vi "ch_to_cellement.vi"(7 "chtree config":T1={"ch"=[{"String"="通道名称", "use"=TRUE, "display"=0, "Enum"=enum."Chname"}, {"String"="使用", "use"=TRUE, "display"=0, "Enum"=enum."USE"}, {"String"="频率", "use"=TRUE, "display"=0, "Enum"=enum."fre"}, {"String"="范围", "use"=FALSE, "display"=0, "Enum"=enum."range"}, {"String"="传感器", "use"=TRUE, "display"=0, "Enum"=enum."senNO"}, {"String"="物理量", "use"=TRUE, "display"=0, "Enum"=enum."PHname"}, {"String"="单位", "use"=TRUE, "display"=0, "Enum"=enum."unit"}, {"String"="校准类型", "use"=FALSE, "display"=0, "Enum"=enum."CALclass"}, {"String"="校准系数", "use"=FALSE, "display"=0, "Enum"=enum."K"}, {"String"="校准偏量", "use"=TRUE, "display"=0, "Enum"=enum."K"}, {"String"="报警", "use"=TRUE, "display"=0, "Enum"=enum."Alrm"}, {"String"="", "use"=FALSE, "display"=0, "Enum"=enum."CNO."}, {"String"="", "use"=FALSE, "display"=0, "Enum"=enum."CNO."}], "displya num"=1, "range value"=["0~10V", "0~5V", "±10V", "±5V", "", "", "", "", "", "", "", "", "", "", "", "", "", "", "", ""], "Etype"=["电压", "电流", "电阻", "±5V", "", "", "", "", "", "", "", "", "", "", "", "", "", "", "", ""], "CLASS"=[]}, 10 "element":T3 {"display" format="%b"}) -> (2 "chtree cell Array":string[](array[string]))   [LabVIEW 2011]
uses:
  singlechtype.ctl
  chtype.ctl
  config table enum.ctl
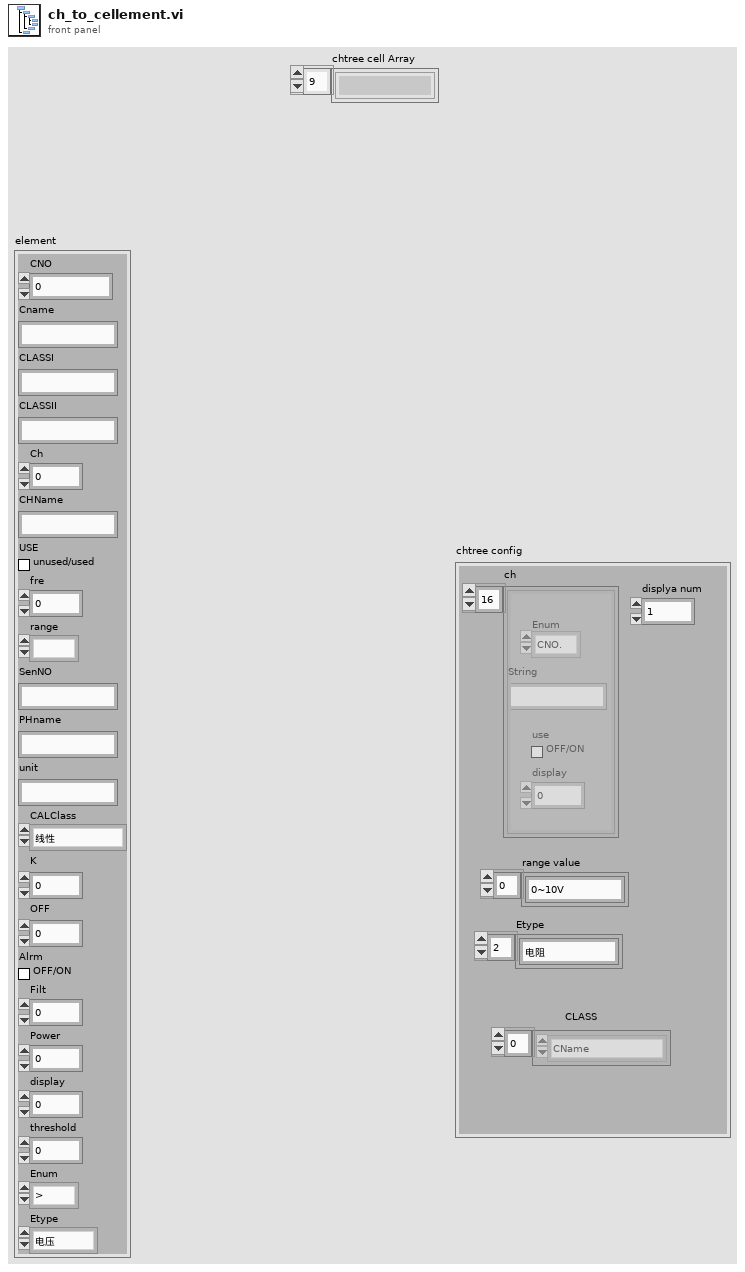
[diagram p1: front panel]
types:
  T1 = typedef "chtype.ctl" = cluster{"ch":cluster{"String":string, "use":bool, "display":u16, "Enum":T2}[], "displya num":i32, "range value":string[], "Etype":string[], "CLASS":enum16{"CName", "CNO", "ClassI", "ClassII"}[]}
  T2 = typedef "config table enum.ctl" = enum16{"CNO.", "CName", "CLASSI", "CLASSII", "ch", "Chname", "USE", "fre", "range", "senNO", "PHname", "unit", "CALclass", "K", "OFF", "Alrm", "filt", "Power", "display", "threshold", "compare", "Etype"}
  T3 = typedef "singlechtype.ctl" = cluster{"CNO":u8, "Cname":string, "CLASSI":string, "CLASSII":string, "Ch":u8, "CHName":string, "USE":bool, "fre":dbl, "range":enum16{""}, "SenNO":string, "PHname":string, "unit":string, "CALClass":enum8{"线性", "查表", "公式"}, "K":dbl, "OFF":dbl, "Alrm":bool, "Filt":dbl, "Power":u8, "display":u8, "threshold ":dbl, "Enum":enum16{">", ">=", "<", "<=", "<>(在范围内）", "><（在范围外）"}, "Etype":enum16{"电压", "电流", "电阻", "热电偶K", "热电偶T"}}
  T4 = cluster{"String":string, "use":bool, "display":u16, "Enum":T2}[]
  T5 = enum16{">", ">=", "<", "<=", "<>(在范围内）", "><（在范围外）"}
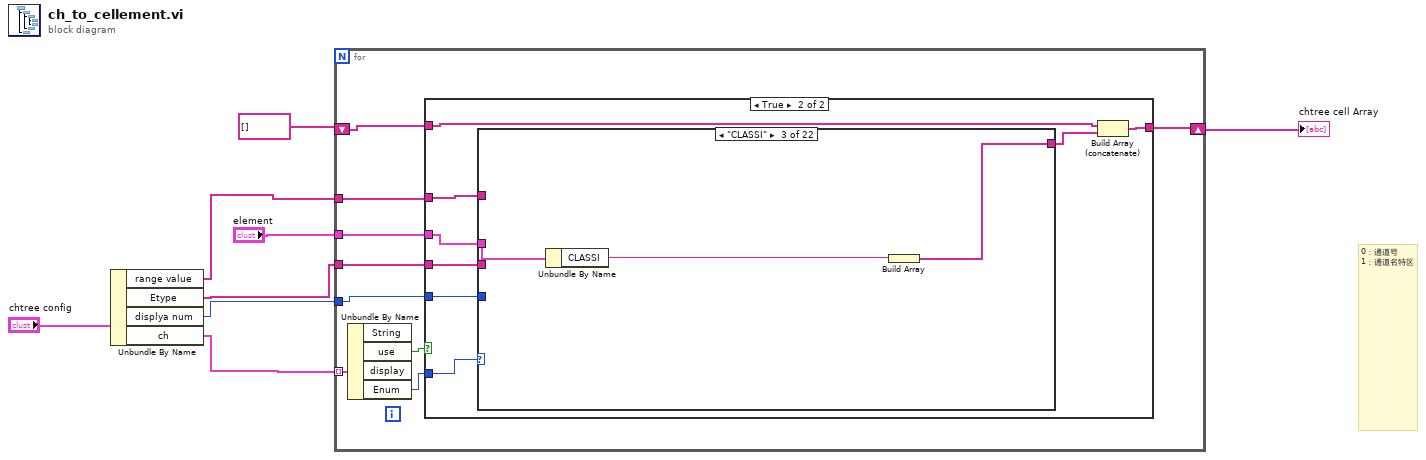
[diagram p0: block diagram]
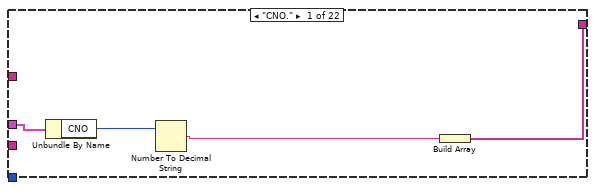
[diagram p3: hidden frame]
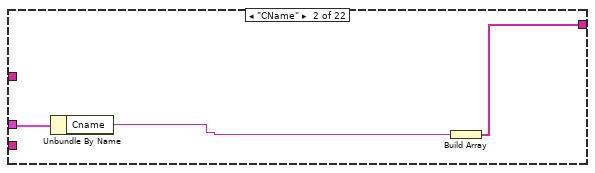
[diagram p4: hidden frame]
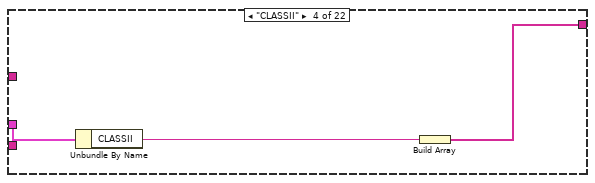
[diagram p5: hidden frame]
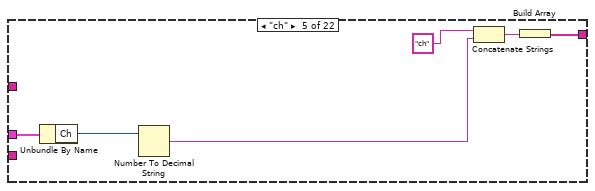
[diagram p6: hidden frame]
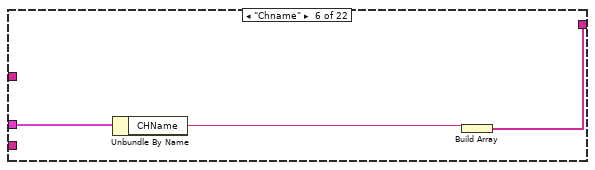
[diagram p7: hidden frame]
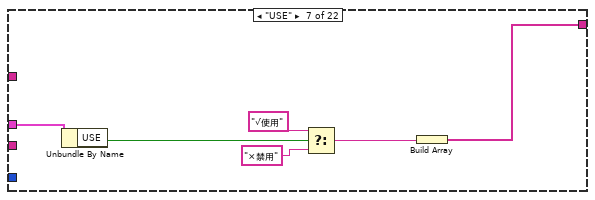
[diagram p8: hidden frame]
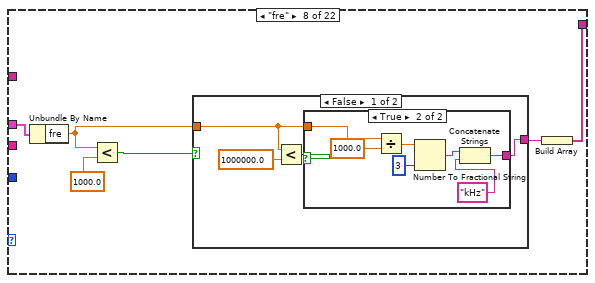
[diagram p9: hidden frame]
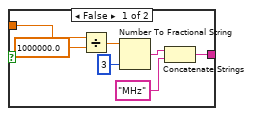
[diagram p10: hidden frame]
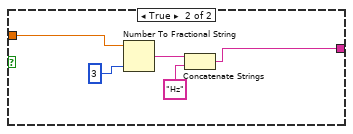
[diagram p11: hidden frame]
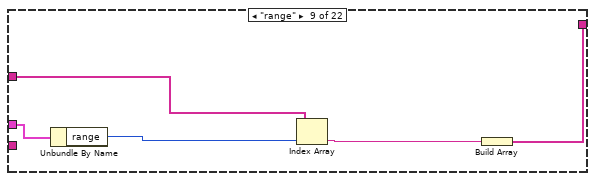
[diagram p12: hidden frame]
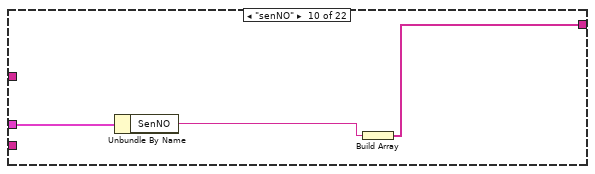
[diagram p13: hidden frame]
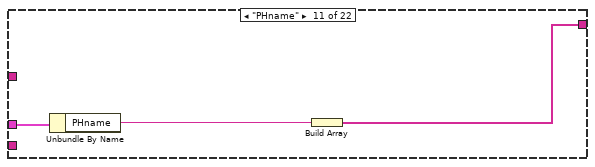
[diagram p14: hidden frame]
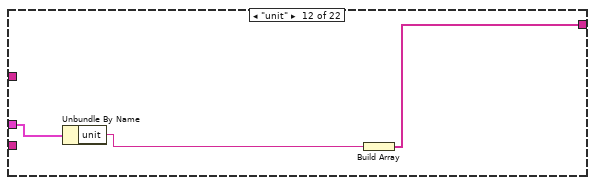
[diagram p15: hidden frame]
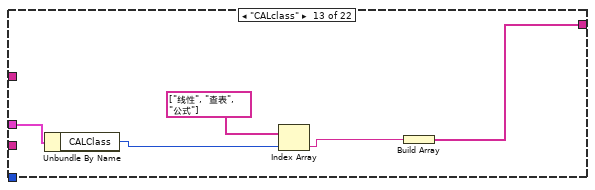
[diagram p16: hidden frame]
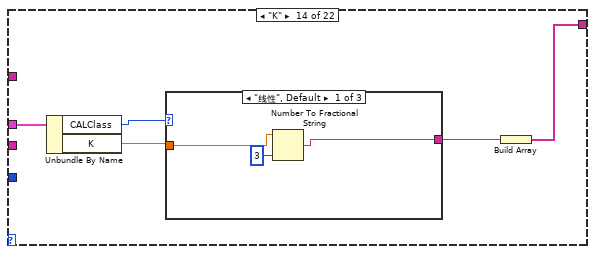
[diagram p17: hidden frame]
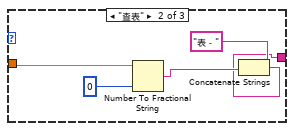
[diagram p18: hidden frame]
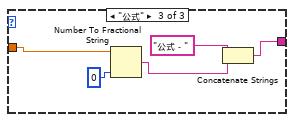
[diagram p19: hidden frame]
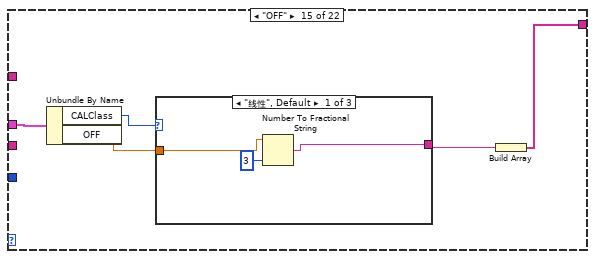
[diagram p20: hidden frame]
diagram:
  # "0：通道号\n1：通道名特区"
  n1 = Unbundle By Name("chtree config") -> ("range value"=w2:string[], "Etype"=w1:string[], "displya num"=w4:i32, "ch"=w5:T4)
  n2 = for {
    tunnel: "element" -> [w15]
    shift-right: [w16] -> w3
    shift-left: string[] [] -> [w17]
    tunnel: w5 -> [w14] mode=indexing
    tunnel: w2 -> [w13]
    tunnel: w4 -> [w12]
    tunnel: w1 -> [w9]
    n3 = Unbundle By Name(w14) -> ("use"=w10:bool, "Enum"=w11:T2)  [unwired: 2 out]
    n4 = case shown="True" w10 {
      tunnel: w17 -> [w18 w26]
      tunnel: [w18 w23] -> w16
      tunnel: w15 -> [_ w25]
      tunnel: w11 -> [_ w22]
      tunnel: w13 -> [_ w21]
      tunnel: w12 -> [_ w20]
      tunnel: w9 -> [_ w19]
      frame False {
      }
      frame True {
        n5 = case shown="\"CLASSI\"" w22 {
          tunnel: w25 -> [w29 w33 w36 w39 w45 w48 w54 w60 w88 w91 w94 w97 w102 w107 w125 w144 w149 w182 w192 w201 w205 w216]
          tunnel: [w28 w31 w34 w37 w40 w47 w49 w55 w87 w89 w92 w95 w101 w103 w121 w140 w145 w178 w189 w198 w204 w213] -> w24
          tunnel: w21 -> [_ _ _ _ _ _ _ _ w84 _ _ _ _ _ _ _ _ _ _ _ _ _]
          tunnel: w20 -> [_ _ _ _ _ _ _ _ _ _ _ _ _ _ _ _ _ _ w188 _ _ _]
          tunnel: w19 -> [_ _ _ _ _ _ _ _ _ _ _ _ _ _ _ _ _ _ _ _ _ w212]
          frame "CNO." {
            n6 = Unbundle By Name(w29) -> ("CNO"=w30:u8)
            n7 = Number To Decimal String(number=w30) -> (decimal integer string=w27:string)  [unwired: 1 in]
            n8 = Build Array(w27) -> (w28:string[])
          }
          frame "CName" {
            n9 = Unbundle By Name(w33) -> ("Cname"=w32:string)
            n10 = Build Array(w32) -> (w31:string[])
          }
          frame "CLASSI" {
            n11 = Unbundle By Name(w36) -> ("CLASSI"=w35:string)
            n12 = Build Array(w35) -> (w34:string[])
          }
          frame "CLASSII" {
            n13 = Unbundle By Name(w39) -> ("CLASSII"=w38:string)
            n14 = Build Array(w38) -> (w37:string[])
          }
          frame "ch" {
            n15 = Unbundle By Name(w45) -> ("Ch"=w44:u8)
            n16 = Number To Decimal String(number=w44) -> (decimal integer string=w43:string)  [unwired: 1 in]
            n17 = Concatenate Strings("ch", w43) -> (w41:string)
            n18 = Build Array(w41) -> (w40:string[])
          }
          frame "Chname" {
            n19 = Unbundle By Name(w48) -> ("CHName"=w46:string)
            n20 = Build Array(w46) -> (w47:string[])
          }
          frame "USE" {
            n21 = Unbundle By Name(w54) -> ("USE"=w53:bool)
            n22 = Select(t="√使用", s=w53, f="×禁用") -> (s? t:f=w50:string)
            n23 = Build Array(w50) -> (w49:string[])
          }
          frame "fre" {
            n24 = Unbundle By Name(w60) -> ("fre"=w57:dbl)
            n25 = Less?(x=w57, y=1000.0) -> (x < y?=w58:bool)
            n26 = case shown="False" w58 {
              tunnel: w57 -> [w62 w83]
              tunnel: [w61 w79] -> w56
              frame False {
                n27 = Less?(x=w62, y=1000000.0) -> (x < y?=w63:bool)
                n28 = case shown="True" w63 {
                  tunnel: w62 -> [w71 w78]
                  tunnel: [w65 w72] -> w61
                  frame False {
                    n29 = Divide(x=w71, y=1000000.0) -> (x/y=w69:dbl)
                    n30 = Number To Fractional String(number=w69, precision (6)=i16 3) -> (F-format string=w67:string)  [unwired: 2 in]
                    n31 = Concatenate Strings(w67, "MHz") -> (w65:string)
                  }
                  frame True {
                    n32 = Divide(x=w78, y=1000.0) -> (x/y=w76:dbl)
                    n33 = Number To Fractional String(number=w76, precision (6)=i16 3) -> (F-format string=w74:string)  [unwired: 2 in]
                    n34 = Concatenate Strings(w74, "kHz") -> (w72:string)
                  }
                }
              }
              frame True {
                n35 = Number To Fractional String(number=w83, precision (6)=i16 3) -> (F-format string=w81:string)  [unwired: 2 in]
                n36 = Concatenate Strings(w81, "Hz") -> (w79:string)
              }
            }
            n37 = Build Array(w56) -> (w55:string[])
          }
          frame "range" {
            n38 = Unbundle By Name(w88) -> ("range"=w85:enum16{""})
            n39 = Index Array(array=w84, index=w85) -> (element=w86:string)
            n40 = Build Array(w86) -> (w87:string[])
          }
          frame "senNO" {
            n41 = Unbundle By Name(w91) -> ("SenNO"=w90:string)
            n42 = Build Array(w90) -> (w89:string[])
          }
          frame "PHname" {
            n43 = Unbundle By Name(w94) -> ("PHname"=w93:string)
            n44 = Build Array(w93) -> (w92:string[])
          }
          frame "unit" {
            n45 = Unbundle By Name(w97) -> ("unit"=w96:string)
            n46 = Build Array(w96) -> (w95:string[])
          }
          frame "CALclass" {
            n47 = Unbundle By Name(w102) -> ("CALClass"=w99:enum8{"线性", "查表", "公式"})
            n48 = Index Array(array=string[] ["线性", "查表", "公式"], index=w99) -> (element=w98:string)
            n49 = Build Array(w98) -> (w101:string[])
          }
          frame "K" {
            n50 = Unbundle By Name(w107) -> ("CALClass"=w106:enum8{"线性", "查表", "公式"}, "K"=w105:dbl)
            n51 = case shown="\"线性\", Default" w106 {
              tunnel: w105 -> [w110 w115 w119]
              tunnel: [w109 w111 w116] -> w104
              frame "线性", Default {
                n52 = Number To Fractional String(number=w110, precision (6)=i16 3) -> (F-format string=w109:string)  [unwired: 2 in]
              }
              frame "查表" {
                n53 = Number To Fractional String(number=w115, precision (6)=i16 0) -> (F-format string=w112:string)  [unwired: 2 in]
                n54 = Concatenate Strings("表－", w112) -> (w111:string)
              }
              frame "公式" {
                n55 = Number To Fractional String(number=w119, precision (6)=i16 0) -> (F-format string=w117:string)  [unwired: 2 in]
                n56 = Concatenate Strings("公式－", w117) -> (w116:string)
              }
            }
            n57 = Build Array(w104) -> (w103:string[])
          }
          frame "OFF" {
            n58 = Unbundle By Name(w125) -> ("CALClass"=w123:enum8{"线性", "查表", "公式"}, "OFF"=w124:dbl)
            n59 = case shown="\"线性\", Default" w123 {
              tunnel: w124 -> [w128 w133 w137]
              tunnel: [w127 w129 w134] -> w122
              frame "线性", Default {
                n60 = Number To Fractional String(number=w128, precision (6)=i16 3) -> (F-format string=w127:string)  [unwired: 2 in]
              }
              frame "查表" {
                n61 = Number To Fractional String(number=w133, precision (6)=i16 0) -> (F-format string=w130:string)  [unwired: 2 in]
                n62 = Concatenate Strings("表－", w130) -> (w129:string)
              }
              frame "公式" {
                n63 = Number To Fractional String(number=w137, precision (6)=i16 0) -> (F-format string=w135:string)  [unwired: 2 in]
                n64 = Concatenate Strings("公式－", w135) -> (w134:string)
              }
            }
            n65 = Build Array(w122) -> (w121:string[])
          }
          frame "Alrm" {
            n66 = Unbundle By Name(w144) -> ("Alrm"=w142:bool)
            n67 = Select(t="警告", s=w142, f="不报警") -> (s? t:f=w141:string)
            n68 = Build Array(w141) -> (w140:string[])
          }
          frame "filt" {
            n69 = Unbundle By Name(w149) -> ("Filt"=w147:dbl)
            n70 = Less Or Equal To 0?(x=w147) -> (x <= 0?=w148:bool)
            n71 = case shown="False" w148 {
              tunnel: [w150 "不滤波"] -> w146
              tunnel: w147 -> [w151 _]
              frame False {
                n72 = Less?(x=w151, y=1000.0) -> (x < y?=w152:bool)
                n73 = case shown="True" w152 {
                  tunnel: w151 -> [w155 w176]
                  tunnel: [w154 w172] -> w150
                  frame False {
                    n74 = Less?(x=w155, y=1000000.0) -> (x < y?=w156:bool)
                    n75 = case shown="False" w156 {
                      tunnel: w155 -> [w164 w171]
                      tunnel: [w158 w165] -> w154
                      frame False {
                        n76 = Divide(x=w164, y=1000000.0) -> (x/y=w162:dbl)
                        n77 = Number To Fractional String(number=w162, precision (6)=i16 3) -> (F-format string=w160:string)  [unwired: 2 in]
                        n78 = Concatenate Strings(w160, "MHz") -> (w158:string)
                      }
                      frame True {
                        n79 = Divide(x=w171, y=1000.0) -> (x/y=w169:dbl)
                        n80 = Number To Fractional String(number=w169, precision (6)=i16 3) -> (F-format string=w167:string)  [unwired: 2 in]
                        n81 = Concatenate Strings(w167, "kHz") -> (w165:string)
                      }
                    }
                  }
                  frame True {
                    n82 = Number To Fractional String(number=w176, precision (6)=i16 3) -> (F-format string=w174:string)  [unwired: 2 in]
                    n83 = Concatenate Strings(w174, "Hz") -> (w172:string)
                  }
                }
              }
              frame True {
              }
            }
            n84 = Build Array(w146) -> (w145:string[])
          }
          frame "Power", Default {
            n85 = Unbundle By Name(w182) -> ("Power"=w180:u8)
            n86 = Equal To 0?(x=w180) -> (x = 0?=w181:bool)
            n87 = case shown="False" w181 {
              tunnel: [w185 "禁止供电"] -> w179
              tunnel: w180 -> [w186 _]
              frame False {
                n88 = Number To Decimal String(number=w186) -> (decimal integer string=w184:string)  [unwired: 1 in]
                n89 = Concatenate Strings(w184, "V") -> (w185:string)
              }
              frame True {
              }
            }
            n90 = Build Array(w179) -> (w178:string[])
          }
          frame "display" {
            n91 = Unbundle By Name(w192) -> ("display"=w191:u8)
            n92 = Number To Boolean Array(number=w191) -> (Boolean array=w190:bool[])
            n93 = for {
              N: w188 -> [_]
              tunnel: w190 -> [w196] mode=indexing
              tunnel: [w194] -> w189 mode=indexing
              tunnel: [w194] -> _ mode=indexing
              n94 = Select(t="√", s=w196, f="×") -> (s? t:f=w194:string)
            }
          }
          frame "threshold" {
            n95 = Unbundle By Name(w201) -> ("threshold"=w200:dbl)
            n96 = Number To Fractional String(number=w200, precision (6)=i16 3) -> (F-format string=w197:string)  [unwired: 2 in]
            n97 = Build Array(w197) -> (w198:string[])
          }
          frame "compare" {
            n98 = Unbundle By Name(w205) -> ("Enum"=w202:T5)
            n99 = case shown="\">\", Default" w202 {
              tunnel: [">" "≥" "＜" "≤" "<>" "><"] -> w203
              frame ">", Default {
              }
              frame ">=" {
              }
              frame "<" {
              }
              frame "<=" {
              }
              frame "<>(在范围内）" {
              }
              frame "><（在范围外）" {
              }
            }
            n100 = Build Array(w203) -> (w204:string[])
          }
          frame "Etype" {
            n101 = Unbundle By Name(w216) -> ("Etype"=w215:enum16{"电压", "电流", "电阻", "热电偶K", "热电偶T"})
            n102 = Index Array(array=w212, index=w215) -> (element=w214:string)
            n103 = Build Array(w214) -> (w213:string[])
          }
        }
        n104 = Build Array (concatenate)(w26, w24) -> (w23:string[])
      }
    }
  }
  "chtree cell Array" <- w3
